vi "get new coefficients.vi"(2 "lamda":dbl format="%0.2e", 3 "Beta":dbl[](array[numeric]) format="%0.2f", 4 "Alpha":dbl[][](array[numeric]) format="%0.2f", 5 "Coefficients":dbl[](array[numeric]) format="%0.2f") -> (0 "error":i32, 1 "New Coefficients":dbl[](array[numeric]) format="%0.2f")   [LabVIEW 2017, in "NI_AALPro.lvlib"]
uses:
  <vilib>/Analysis/NI_AALPro.lvlib
  <resource>/lvanlys.dll
panel:
  # "Get New Coefficients"
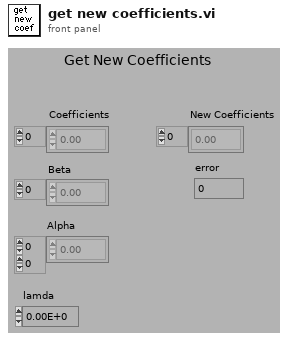
[diagram p1: front panel]
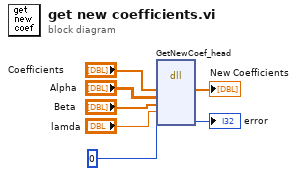
[diagram p0: block diagram]
diagram:
  n1 = dll-call lib="e:/builds/penguin/labview/branches/2017/dev/dist/resource/lvanlys.*" fn="GetNewCoef_head"("Coefficients"="Coefficients", "Alpha"="Alpha", "Beta"="Beta", "lamda"="lamda", 0) -> ("Coefficients"=→"New Coefficients":dbl[], →"error":i32)  [unwired: 7 in, 2 out]
